vi "GetPathPointsAndActions.vi"(8 "error in":T2) -> (0 "error out":T2, 1 "CoordY":sgl[](array[numeric]), 2 "CoordX":sgl[](array[numeric]), 3 "Actionlist":T1[](array[typedef]) items=["Manual Handshake", "Z Spectroscopy", "DAC Spectroscopy", "Low Frequency Spectroscopy", "External Spectroscopy", "Move Z to Home", "Z Approach"], 5 "PathPoints":string[][](table))   [LabVIEW 2016]
doc: "This VI provides information about the path mode. The outputs are:\n- PathPoints: 2D-Array of strings which can be connected to a LabVIEW table indicator. It contains all path points that has been set since the daisy server had been started and shows them clearly in a table.\n- Actionlist: 1D-Array that contains all actions, which has been set.\n- CoordX: 1D-Array of floats with all X coordinates of all set path points\n- CoordY: 1D-Array of floats with all Y coordinates of all set path points\nNote that if you defined a grid of points with definegrid.vi, this VI will provide the three points, that are necessary to define the grid in the output variables."
uses:
  Controls/Error_Out.ctl
  Controls/Pathmode-Action_Selection.ctl
  Files_ASC500/DLL/ASC500_RemoteControlV27.dll
panel:
  out "Actionnumbers":sgl[](array[numeric])
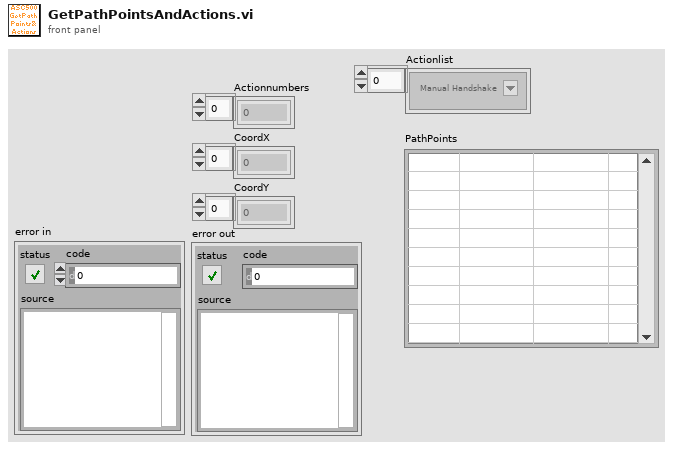
[diagram p1: front panel]
types:
  T1 = typedef "Pathmode-Action_Selection.ctl" = i32
  T2 = typedef "Error_Out.ctl" = errorcluster
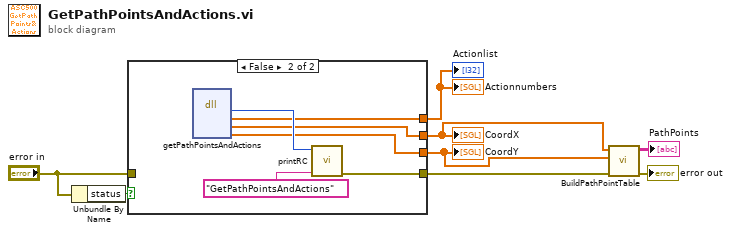
[diagram p0: block diagram]
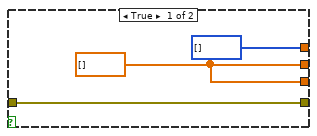
[diagram p2: hidden frame]
diagram:
  n1 = Unbundle By Name("error in") -> ("status"=w7:bool)
  n2 = case shown="False" w7 {
    tunnel: "error in" -> [w11 _]
    tunnel: [w11 w16] -> w2
    tunnel: [i32[] [] ("Actionnumbers") w14] -> w6
    tunnel: [w9 w13] -> w4
    tunnel: [w9 w12] -> w5
    frame True {
      w9 = sgl[] [] ("CoordX")
    }
    frame False {
      n3 = dll-call lib="G:/SCMOperations/Share/ELE/Produkt Information/ASC500/04 Remote Control/02 development versions/2018Nov06/Files_ASC500/DLL/ASC500_RemoteControlV27.dll" fn="getPathPointsAndActions"() -> ("return type"=w15:i32, "Actionnumbers"=w14:sgl[], "CoordX"=w13:sgl[], "CoordY"=w12:sgl[])  [unwired: 6 in, 2 out]
      n4 = call "printRC.vi"("additional information"="GetPathPointsAndActions", "RC"=w15) -> ("error out"=w16:T2)  [unwired: 9 in]
    }
  }
  "Actionnumbers" <- w6
  "CoordX" <- w4
  "CoordY" <- w5
  "Actionlist" <- w6
  n5 = call "BuildPathPointTable.vi"("error in"=w2, "yCoordinates"=w5, "xCoordinates"=w4) -> ("error out"=→"error out":T2, "PathPoints"=→"PathPoints":string[][])  [unwired: 7 in]
